vi "02_EventStructure3.vi"() -> ()   [LabVIEW 2019]
panel:
  in  "Stop":bool
  out "Lamp2":bool
  out "Lamp1":bool
  in  "Button":bool
  out "Numeric":i32
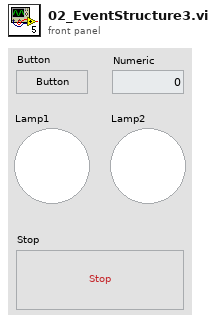
[diagram p1: front panel]
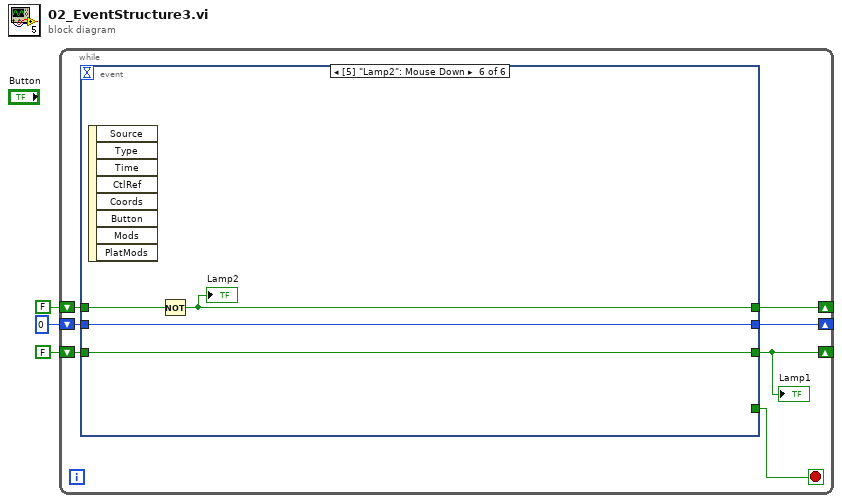
[diagram p0: block diagram]
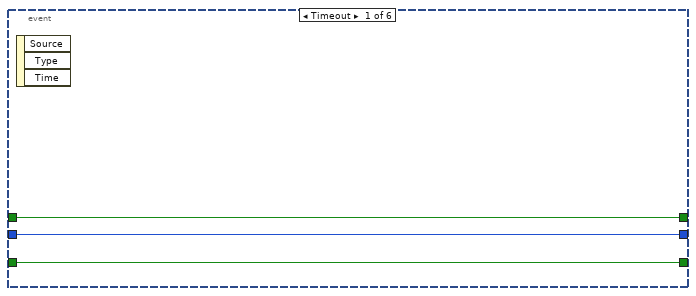
[diagram p2: hidden frame]
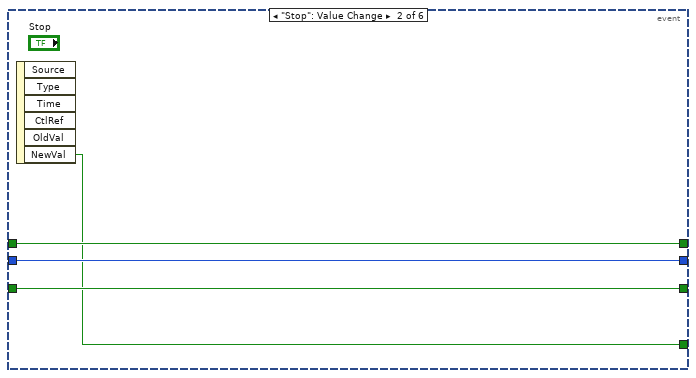
[diagram p3: hidden frame]
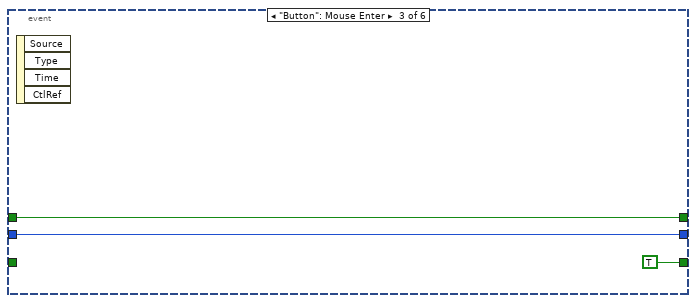
[diagram p4: hidden frame]
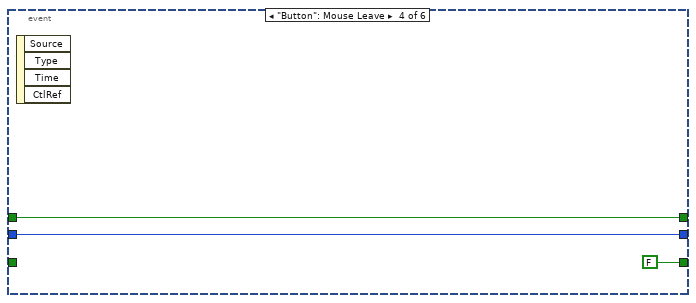
[diagram p5: hidden frame]
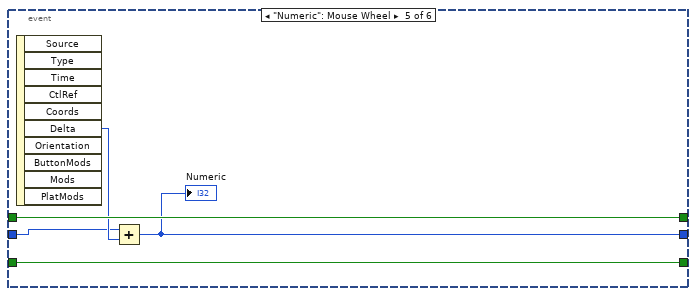
[diagram p6: hidden frame]
diagram:
  n1 = while {
    shift-right: [w9] -> _
    shift-left: FALSE -> [w10]
    shift-right: [w7] -> _
    shift-left: 0 -> [w6]
    shift-right: [w5] -> _
    shift-left: FALSE -> [w4]
    stop <- w8 stop-if-true
    n2 = event shown="[5] \"Lamp2\": Mouse Down" {
      selector: _ -> [_ _ _ _ _ _]
      dyn-events: _ -> [_ _ _ _ _ _]
      timeout: _ -> [_ _ _ _ _ _]
      tunnel: [w13 w17 TRUE FALSE w27 w32] -> w9
      tunnel: w10 -> [w13 w17 _ _ w27 w32]
      tunnel: [_ w14 _ _ _ _] -> w8
      tunnel: [w12 w16 w19 w22 w24 w31] -> w7
      tunnel: w6 -> [w12 w16 w19 w22 w25 w31]
      tunnel: [w11 w15 w18 w21 w28 w29] -> w5
      tunnel: w4 -> [w11 w15 w18 w21 w28 w30]
      event Timeout {
        n3 = event-data() -> ()  [unwired: 1 in, 3 out]
      }
      event "Stop": Value Change {
        n4 = event-data() -> ("NewVal"=w14:bool)  [unwired: 1 in, 5 out]
      }
      event "Button": Mouse Enter {
        n5 = event-data() -> ()  [unwired: 1 in, 4 out]
      }
      event "Button": Mouse Leave {
        n6 = event-data() -> ()  [unwired: 1 in, 4 out]
      }
      event "Numeric": Mouse Wheel {
        n7 = event-data() -> ("Delta"=w26:i32)  [unwired: 1 in, 9 out]
        n8 = Add(x=w25, y=w26) -> (x+y=w24:i32)
        "Numeric" <- w24
      }
      event "Lamp2": Mouse Down {
        n9 = event-data() -> ()  [unwired: 1 in, 8 out]
        n10 = Not(x=w30) -> (.not. x?=w29:bool)
        "Lamp2" <- w29
      }
    }
    "Lamp1" <- w9
  }
